vi "TraverseControl_High.vi"(0 "Mode":T3=enum."Read traverse position", 1 "Route Checking?":bool, 2 "Home":T2, 3 "Traverse Name":string, 5 "Extra command String":string, 6 "Work in Tunnel Coordinates":T1, 7 "Model       Roll      Pitch       Yaw (deg)":sgl[](array[numeric]) format="%#.2f", 9 "Final iteration of 3D_Trav Loop":bool=TRUE, 11 "Position input XYZ":sgl[](array[numeric])=[0.0, 0.0, 0.0] format="%.2f", 12 "Last Part of Move?":bool, 13 "Speed Factor":sgl=1.0 min=0.1 max=5 format="%.2f", 14 "Backlash Compensation?":bool=TRUE) -> (4 "Position Output XYZ":sgl[](array[numeric]) format="%.2f", 15 "Error String":string)   [LabVIEW 2017]
uses:
  Anemometry/Anemometry Sub Vis/Gen Trav/Trav_mode.ctl
  Anemometry/Anemometry Sub Vis/Controls/Home.ctl
  Anemometry/Anemometry Sub Vis/Controls/Tunnel_Coordinates.ctl
  Anemometry/Anemometry Sub Vis/Globals/Extra_Commands_Global.vi
  Anemometry/Anemometry Sub Vis/Globals/Trav_pos_global.vi
  Anemometry/Anemometry Sub Vis/Gen Trav/Route mapping/Route_mapping_global.vi
panel:
  out "Offset Array":sgl[](array[numeric])
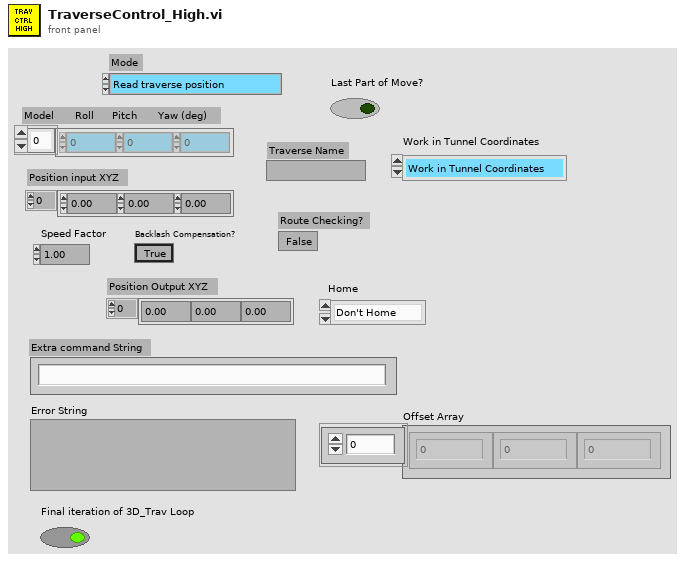
[diagram p1: front panel]
types:
  T1 = typedef "Tunnel_Coordinates.ctl" = enum16{"Work in Tunnel Coordinates", "Work in Model Coordinates"}
  T2 = typedef "Home.ctl" = enum16{"Don't Home", "Home  +X", "Home  -X", "Home  +Y", "Home  -Y", "Home  +Z", "Home  -Z"}
  T3 = typedef "Trav_mode.ctl" = enum16{"Move traverse", "Read traverse position", "Teach Position"}
  T4 = enum16{"To Traverse Coordinates", "To User Coordinates"}
  T5 = typedef "Axis.ctl" = enum16{"X Axis", "X Axis -ve", "Y Axis", "Y Axis -ve", "Z Axis", "Z Axis -ve"}
  T6 = typedef "Box_size.ctl" = cluster{"Max":sgl, "Min":sgl}[]
  T7 = typedef "Exclude_cluster.ctl" = cluster{"Sizes":T6, "Name":string, "Exclude Type":T8}
  T8 = typedef "Exclusion_type.ctl" = enum16{"Exclude completely", "Allow only vertical moves"}
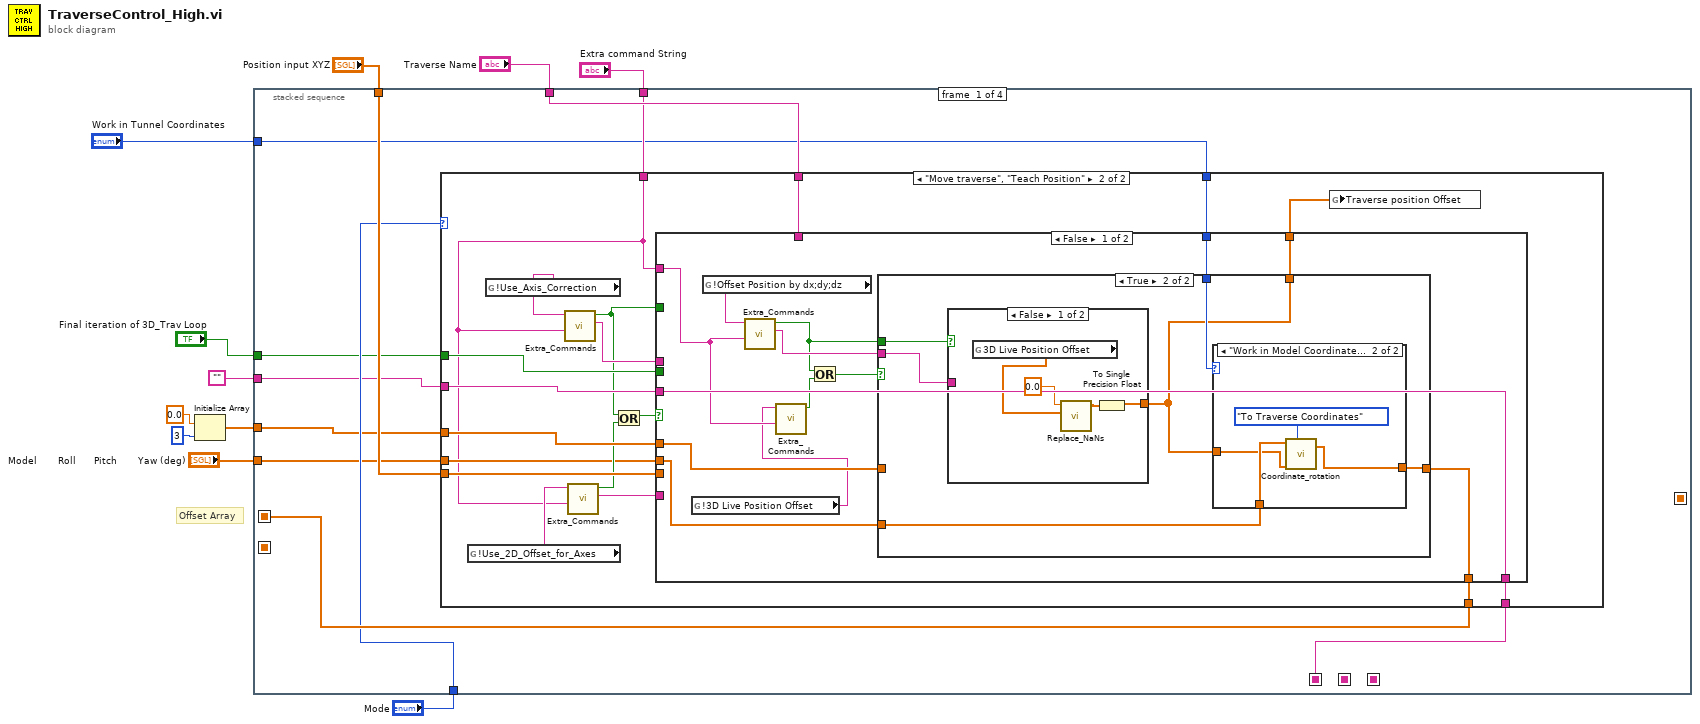
[diagram p0: block diagram]
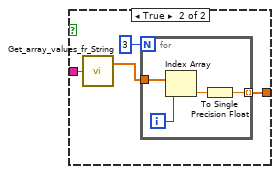
[diagram p4: hidden frame]
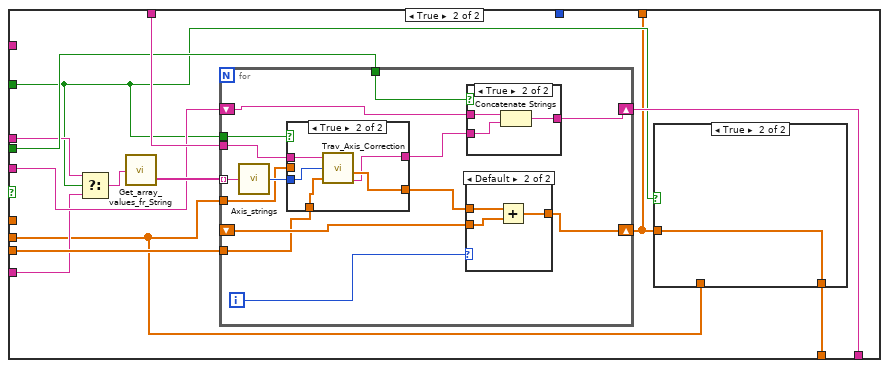
[diagram p6: hidden frame]
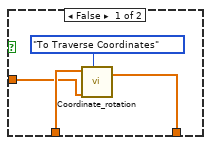
[diagram p7: hidden frame]
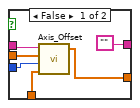
[diagram p8: hidden frame]
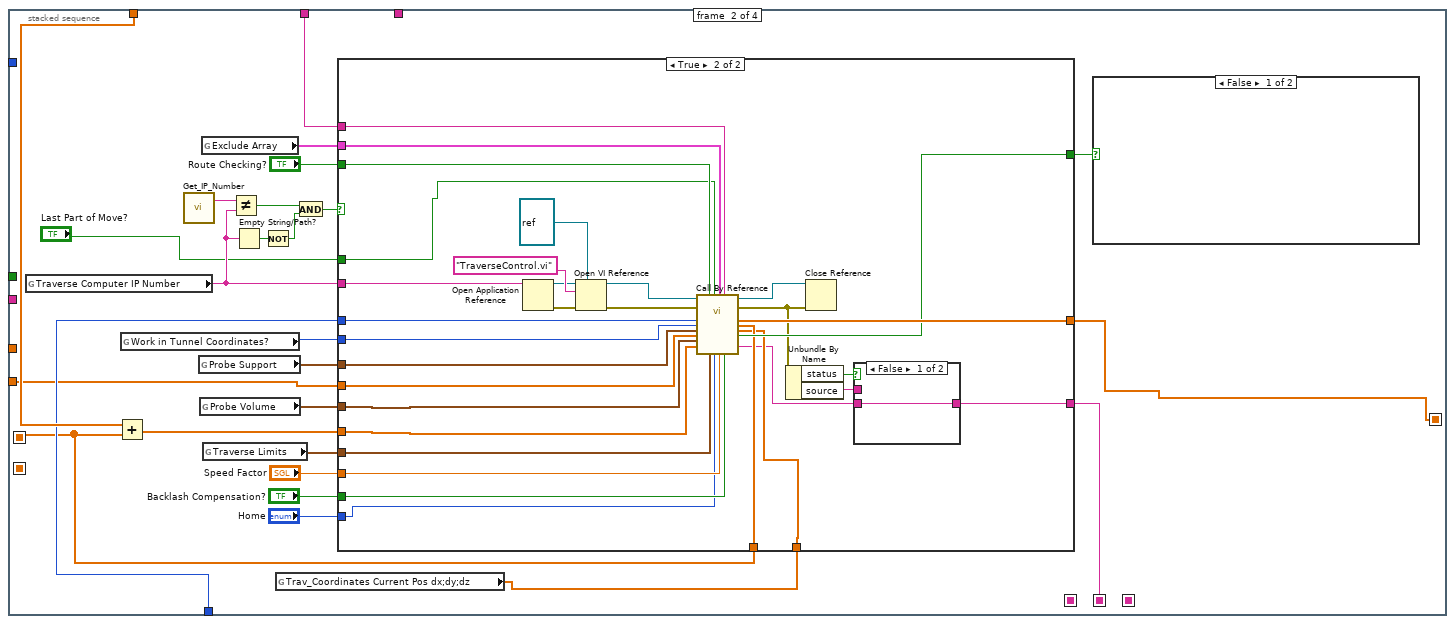
[diagram p11: hidden frame]
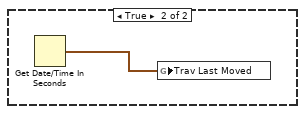
[diagram p12: hidden frame]
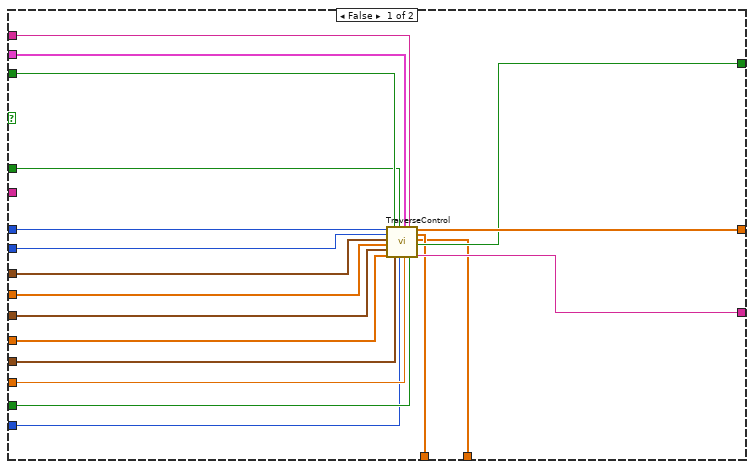
[diagram p13: hidden frame]
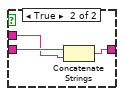
[diagram p14: hidden frame]
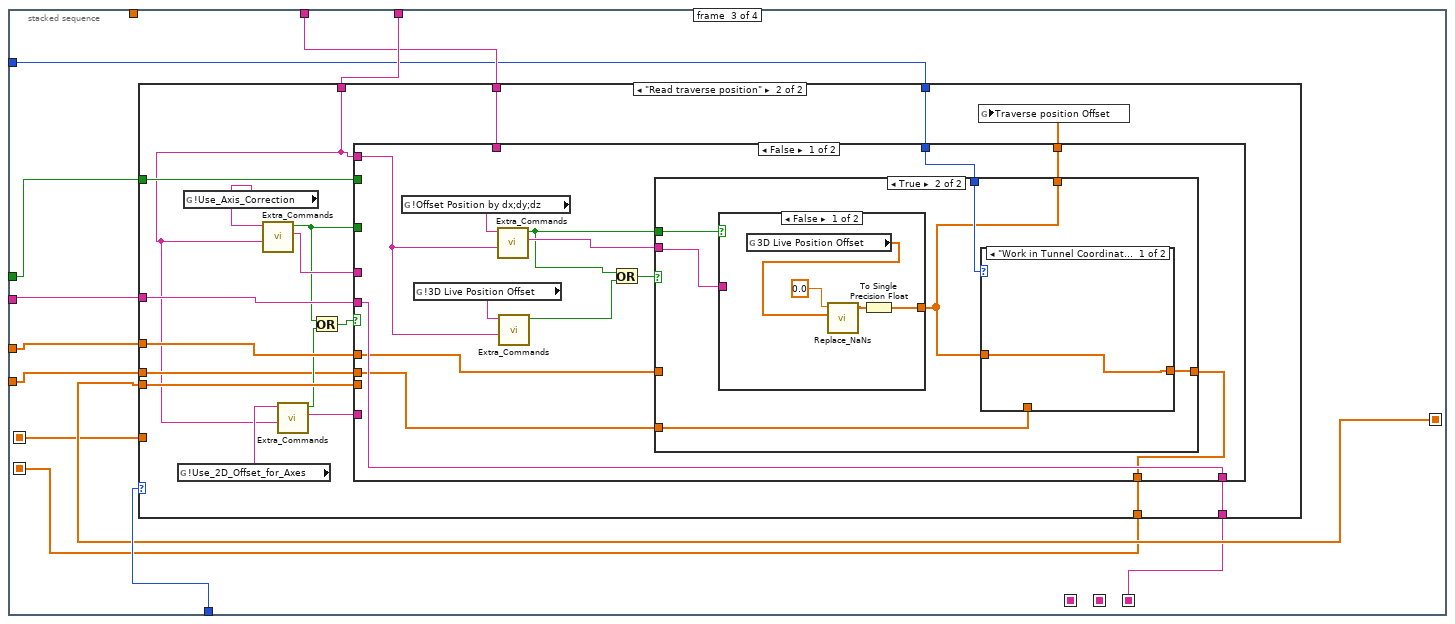
[diagram p15: hidden frame]
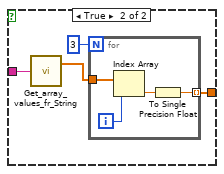
[diagram p18: hidden frame]
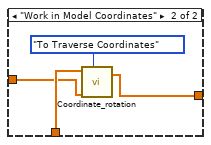
[diagram p19: hidden frame]
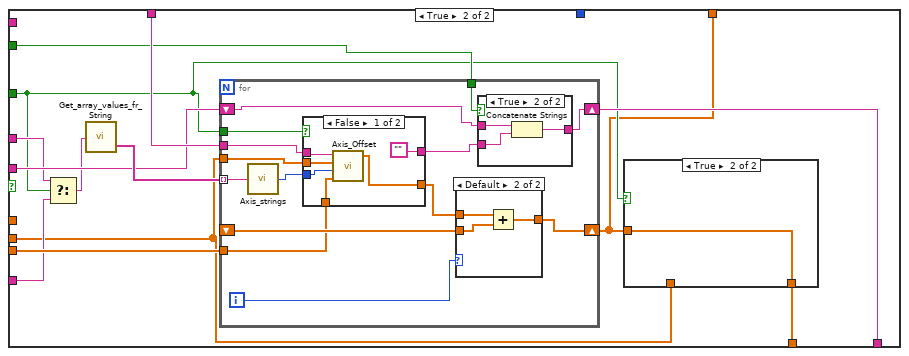
[diagram p20: hidden frame]
diagram:
  # "Offset Array"
  n1 = Initialize Array(sgl 0.0, 3 ("dimension size")) -> (w5:sgl[])
  n2 = stacked-sequence {
    seq-local: [_ w140 _ _] -> [_ _ w219 w337]
    seq-local: [w22 _ _ _] -> [_ w132 w215 _]
    seq-local: [w19 _ _ _] -> [_ _ _ w333]
    seq-local: [_ _ w217 _] -> [_ _ _ w332]
    seq-local: [_ _ w216 _] -> [_ _ _ w335]
    seq-local: [_ w135 _ _] -> [_ _ _ w334]
    tunnel: "Traverse Name" -> [w21 w139 w221 _]
    tunnel: "Position input XYZ" -> [w20 w138 _ _]
    tunnel: "Mode" -> [w17 w136 w223 _]
    tunnel: "Extra command String" -> [w18 _ w222 _]
    tunnel: w5 -> [w16 _ w218 _]
    tunnel: "" -> [w15 _ w220 _]
    tunnel: "Final iteration of 3D_Trav Loop" -> [w14 _ w214 _]
    tunnel: "Model       Roll      Pitch       Yaw (deg)" -> [w13 w133 w213 _]
    tunnel: "Work in Tunnel Coordinates" -> [w12 _ w212 _]
    frame #0 {
      n3 = case shown="\"Move traverse\", \"Teach Position\"" w17 {
        tunnel: [w23 w41] -> w22
        tunnel: w21 -> [_ w40]
        tunnel: w20 -> [_ w38]
        tunnel: [w24 w37] -> w19
        tunnel: w18 -> [_ w27]
        tunnel: w16 -> [w23 w36]
        tunnel: w15 -> [w24 w35]
        tunnel: w14 -> [_ w34]
        tunnel: w13 -> [_ w28]
        tunnel: w12 -> [_ w25]
        frame Default {
        }
        frame "Move traverse", "Teach Position" {
          n4 = global read "Extra_Commands_Global.vi" "!Use_2D_Offset_for_Axes"() -> (w33:string)
          n5 = global read "Extra_Commands_Global.vi" "!Use_Axis_Correction"() -> (w42:string)
          n6 = call "Extra_Commands.vi"("String to Search"=w27, "Command"=w42) -> ("String Value"=w39:string, "Command Found"=w30:bool)  [unwired: 1 in, 3 out]
          n7 = call "Extra_Commands.vi"("String to Search"=w27, "Command"=w33) -> ("String Value"=w29:string, "Command Found"=w32:bool)  [unwired: 1 in, 3 out]
          n8 = Or(x=w30, y=w32) -> (x .or. y?=w31:bool)
          n9 = case shown="False" w31 {
            tunnel: [w51 w82] -> w41
            tunnel: w38 -> [_ w90]
            tunnel: w40 -> [_ w91]
            tunnel: w39 -> [_ w86]
            tunnel: [w55 w87] -> w37
            tunnel: w35 -> [w55 w89]
            tunnel: w36 -> [w52 _]
            tunnel: w34 -> [_ w88]
            tunnel: w30 -> [_ w81]
            tunnel: w29 -> [_ w85]
            tunnel: w28 -> [w49 w83]
            tunnel: w27 -> [w44 _]
            tunnel: [w48 w80] -> w26
            tunnel: w25 -> [w50 _]
            frame False {
              n10 = global read "Extra_Commands_Global.vi" "!3D Live Position Offset"() -> (w43:string)
              n11 = global read "Extra_Commands_Global.vi" "!Offset Position by dx;dy;dz"() -> (w54:string)
              n12 = call "Extra_Commands.vi"("String to Search"=w44, "Command"=w54) -> ("String Value"=w53:string, "Command Found"=w45:bool)  [unwired: 1 in, 3 out]
              n13 = call "Extra_Commands.vi"("String to Search"=w44, "Command"=w43) -> ("Command Found"=w47:bool)  [unwired: 1 in, 4 out]
              n14 = Or(x=w45, y=w47) -> (x .or. y?=w46:bool)
              n15 = case shown="True" w46 {
                tunnel: w53 -> [_ w62]
                tunnel: [w56 w60] -> w51
                tunnel: w52 -> [w56 _]
                tunnel: w50 -> [_ w61]
                tunnel: w49 -> [_ w59]
                tunnel: [w56 w58] -> w48
                tunnel: w45 -> [_ w57]
                frame False {
                }
                frame True {
                  n16 = case shown="False" w57 {
                    tunnel: w62 -> [_ w69]
                    tunnel: [w64 w67] -> w58
                    frame False {
                      n17 = global read "Trav_pos_global.vi" "3D Live Position Offset"() -> (w63:sgl[])
                      n18 = call "Replace_NaNs.vi"("Array"=w63, "Replacement"=0.0) -> ("Array Out"=w65:dbl[])  [unwired: 9 in]
                      n19 = To Single Precision Float(number=w65) -> (single precision float=w64:sgl[])
                    }
                    frame True {
                      n20 = call "Get_array_values_fr_String.vi"("String Value"=w69) -> ("Numeric Array"=w68:dbl[])  [unwired: 1 out]
                      n21 = for {
                        N: 3 -> [_]
                        tunnel: w68 -> [w74]
                        tunnel: [w71] -> w67 mode=indexing
                        i -> [w73]
                        n22 = Index Array(array=w74, index=w73) -> (element=w72:dbl)
                        n23 = To Single Precision Float(number=w72) -> (single precision float=w71:sgl)
                      }
                    }
                  }
                  n24 = case shown="\"Work in Model Coordinates\"" w61 {
                    tunnel: w58 -> [w75 w76]
                    tunnel: w59 -> [_ w79]
                    tunnel: [w75 w78] -> w60
                    frame "Work in Tunnel Coordinates" {
                    }
                    frame "Work in Model Coordinates" {
                      n25 = call "Coordinate_rotation.vi"("Roll-Pitch-Yaw"=w79, "Input Position"=w76, "Mode"=T4."To Traverse Coordinates") -> ("Output Position"=w78:sgl[])  [unwired: 2 in, 1 out]
                    }
                  }
                }
              }
            }
            frame True {
              n26 = Select(t=w86, s=w81, f=w85) -> (s? t:f=w84:string)
              n27 = call "Get_array_values_fr_String.vi"("String Value"=w84) -> ("String array"=w92:string[])  [unwired: 1 out]
              n28 = for {
                tunnel: w92 -> [w111] mode=indexing
                tunnel: w91 -> [w104]
                tunnel: w90 -> [w102]
                shift-right: [w109] -> w80
                shift-left: _ -> [w110]
                shift-right: [w106] -> w87
                shift-left: w89 -> [w107]
                tunnel: w88 -> [w105]
                tunnel: w81 -> [w98]
                tunnel: w83 -> [w99]
                i -> [w108]
                n29 = call "Axis_strings.vi"("String"=w111) -> ("Enum"=w103:T5)
                n30 = case shown="True" w98 {
                  tunnel: w104 -> [w116 w122]
                  tunnel: w103 -> [w115 w121]
                  tunnel: w102 -> [w114 w120]
                  tunnel: [w117 w119] -> w101
                  tunnel: ["" w118] -> w100
                  tunnel: w99 -> [w112 _]
                  frame False {
                    n31 = call "Axis_Offset.vi"("Position In"=w114, "Axis"=w115, "Roll-Pitch-Yaw"=w112, "Traverse Name"=w116) -> ("Offset Array"=w117:sgl[])  [unwired: 2 out]
                  }
                  frame True {
                    n32 = call "Trav_Axis_Correction.vi"("Traverse Name"=w122, "Axis"=w121, "Position input XYZ"=w120) -> ("Offset Array"=w119:sgl[], "Error String"=w118:string)  [unwired: 2 out]
                  }
                }
                n33 = case shown="Default" w108 {
                  tunnel: w101 -> [w127 w130]
                  tunnel: w110 -> [_ w129]
                  tunnel: [w127 w128] -> w109
                  frame 0 {
                  }
                  frame Default {
                    n34 = Add(x=w130, y=w129) -> (x+y=w128:sgl[])
                  }
                }
                n35 = case shown="True" w105 {
                  tunnel: w100 -> [_ w126]
                  tunnel: w107 -> [w123 w125]
                  tunnel: [w123 w124] -> w106
                  frame False {
                  }
                  frame True {
                    n36 = Concatenate Strings(w125, w126) -> (w124:string)
                  }
                }
              }
              n37 = case shown="True" w81 {
                tunnel: w80 -> [w93 w97]
                tunnel: w83 -> [w96 _]
                tunnel: [w95 w97] -> w82
                frame False {
                  n38 = call "Coordinate_rotation.vi"("Roll-Pitch-Yaw"=w96, "Input Position"=w93, "Mode"=T4."To Traverse Coordinates") -> ("Output Position"=w95:sgl[])  [unwired: 2 in, 1 out]
                }
                frame True {
                }
              }
            }
          }
          n39 = global write "Trav_pos_global.vi" "Traverse position Offset"(w26) -> ()
        }
      }
    }
    frame #1 {
      n40 = global read "Trav_pos_global.vi" "Traverse Computer IP Number"() -> (w150:string)
      n41 = Add(x=w138, y=w132) -> (x+y=w137:sgl[])
      n42 = global read "Trav_pos_global.vi" "Work in Tunnel Coordinates?"() -> (w144:T1)
      n43 = call "Get_IP_Number.vi"() -> ("IP Number"=w156:string)  [unwired: 1 out]
      n44 = global read "Route_mapping_global.vi" "Probe Support"() -> (w143:T6)
      n45 = global read "Route_mapping_global.vi" "Probe Volume"() -> (w145:T6)
      n46 = global read "Route_mapping_global.vi" "Exclude Array"() -> (w147:T7[])
      n47 = global read "Route_mapping_global.vi" "Traverse Limits"() -> (w146:T6)
      n48 = Not Equal?(x=w156, y=w150) -> (x != y?=w149:bool)
      n49 = Empty String/Path?(string/path=w150) -> (empty?=w152:bool)
      n50 = Not(x=w152) -> (.not. x?=w151:bool)
      n51 = global read "Trav_pos_global.vi" "Trav_Coordinates Current Pos dx;dy;dz"() -> (w131:sgl[])
      n52 = And(x=w149, y=w151) -> (x .and. y?=w148:bool)
      n53 = case shown="True" w148 {
        tunnel: "Route Checking?" -> [w169 w207]
        tunnel: w139 -> [w168 w206]
        tunnel: [w175 w205] -> w140
        tunnel: [w176 w197] -> w135
        tunnel: "Backlash Compensation?" -> [w172 w204]
        tunnel: "Speed Factor" -> [w171 w203]
        tunnel: w137 -> [w174 w202]
        tunnel: w133 -> [w173 w201]
        tunnel: w136 -> [w170 w200]
        tunnel: w150 -> [_ w199]
        tunnel: w147 -> [w167 w198]
        tunnel: w146 -> [w166 w194]
        tunnel: w145 -> [w165 w195]
        tunnel: w144 -> [w164 w196]
        tunnel: w143 -> [w163 w193]
        tunnel: "Last Part of Move?" -> [w162 w192]
        tunnel: "Home" -> [w161 w191]
        tunnel: [w160 w190] -> w141
        tunnel: w132 -> [w159 w189]
        tunnel: w131 -> [w158 w188]
        frame False {
          n54 = call "TraverseControl.vi"("Mode"=w170, "Work in Tunnel Coordinates?"=w164, "Probe Support"=w163, "Model       Roll      Pitch       Yaw (deg)"=w173, "Probe Volume"=w165, "Position input XYZ"=w174, "Route Checking?"=w169, "Entire Space"=w166, "Last Part of Move?"=w162, "Home"=w161, "Exclude Array"=w167, "Speed Factor"=w171, "Traverse Name"=w168, "Backlash Compensation?"=w172, "Trav_Coordinates New Pos dx;dy;dz"=w159, "Trav_Coordinates Current Pos dx;dy;dz"=w158) -> ("Position Output XYZ"=w175:sgl[], "Moved?"=w160:bool, "Error String"=w176:string)  [unwired: 1 in]
        }
        frame True {
          n55 = Open Application Reference(11:w199) -> (0:w181:errorcluster, 3:w182:refnum<vi>)  [unwired: 2 in, 1 out]
          n56 = Open VI Reference(type specifier VI Refnum (for type only)=refnum<vi> refnum ("Scout Server"), application reference (local)=w182, vi path="TraverseControl.vi", error in (no error)=w181) -> (vi reference=w185:refnum<vi>, error out=w184:errorcluster)  [unwired: 2 out]
          n57 = call-by-ref "?"(reference=w185, error in=w184, "Mode"=w200, "Work in Tunnel Coordinates?"=w196, "Probe Support"=w193, "Model       Roll      Pitch       Yaw (deg)"=w201, "Probe Volume"=w195, "Position input XYZ"=w202, "Route Checking?"=w207, "Entire Space"=w194, "Last Part of Move?"=w192, "Home"=w191, "Exclude Array"=w198, "Speed Factor"=w203, "Traverse Name"=w206, "Backlash Compensation?"=w204, "Trav_Coordinates New Pos dx;dy;dz"=w189, "Trav_Coordinates Current Pos dx;dy;dz"=w188) -> (reference out=w183:refnum<vi>, error out=w180:errorcluster, "Position Output XYZ"=w205:sgl[], "Moved?"=w190:bool, "Error String"=w178:string)  [unwired: 1 in]
          n58 = Unbundle By Name(w180) -> ("status"=w179:bool, "source"=w177:string)
          n59 = Close Reference(reference=w183, error in (no error)=w180) -> ()  [unwired: 1 out]
          n60 = case shown="False" w179 {
            tunnel: [w208 w211] -> w197
            tunnel: w178 -> [w208 w210]
            tunnel: w177 -> [_ w209]
            frame False {
            }
            frame True {
              n61 = Concatenate Strings(w210, w209) -> (w211:string)
            }
          }
        }
      }
      n62 = case shown="False" w141 {
        frame False {
        }
        frame True {
          n63 = Get Date/Time In Seconds() -> (seconds since 1Jan1904=w157:timestamp)
          n64 = global write "Trav_pos_global.vi" "Trav Last Moved"(w157) -> ()
        }
      }
    }
    frame #2 {
      n65 = case shown="\"Read traverse position\"" w223 {
        tunnel: [w224 w242] -> w217
        tunnel: w221 -> [_ w241]
        tunnel: w219 -> [_ w239]
        tunnel: [w225 w238] -> w216
        tunnel: w222 -> [_ w228]
        tunnel: w218 -> [_ w237]
        tunnel: w220 -> [w225 w236]
        tunnel: w215 -> [w224 _]
        tunnel: w214 -> [_ w235]
        tunnel: w213 -> [_ w229]
        tunnel: w212 -> [_ w226]
        frame Default {
        }
        frame "Read traverse position" {
          n66 = global read "Extra_Commands_Global.vi" "!Use_2D_Offset_for_Axes"() -> (w234:string)
          n67 = global read "Extra_Commands_Global.vi" "!Use_Axis_Correction"() -> (w243:string)
          n68 = call "Extra_Commands.vi"("String to Search"=w228, "Command"=w243) -> ("String Value"=w240:string, "Command Found"=w231:bool)  [unwired: 1 in, 3 out]
          n69 = call "Extra_Commands.vi"("String to Search"=w228, "Command"=w234) -> ("String Value"=w230:string, "Command Found"=w232:bool)  [unwired: 1 in, 3 out]
          n70 = Or(x=w231, y=w232) -> (x .or. y?=w233:bool)
          n71 = case shown="False" w233 {
            tunnel: [w249 w284] -> w242
            tunnel: w239 -> [_ w291]
            tunnel: w241 -> [_ w292]
            tunnel: w240 -> [_ w287]
            tunnel: [w255 w290] -> w238
            tunnel: w236 -> [w255 w289]
            tunnel: w237 -> [w252 _]
            tunnel: w235 -> [_ w288]
            tunnel: w231 -> [_ w282]
            tunnel: w230 -> [_ w286]
            tunnel: w229 -> [w253 w283]
            tunnel: w228 -> [w247 _]
            tunnel: [w250 w281] -> w227
            tunnel: w226 -> [w251 _]
            frame False {
              n72 = global read "Extra_Commands_Global.vi" "!Offset Position by dx;dy;dz"() -> (w256:string)
              n73 = global read "Extra_Commands_Global.vi" "!3D Live Position Offset"() -> (w248:string)
              n74 = call "Extra_Commands.vi"("String to Search"=w247, "Command"=w256) -> ("String Value"=w254:string, "Command Found"=w244:bool)  [unwired: 1 in, 3 out]
              n75 = call "Extra_Commands.vi"("String to Search"=w247, "Command"=w248) -> ("Command Found"=w245:bool)  [unwired: 1 in, 4 out]
              n76 = Or(x=w244, y=w245) -> (x .or. y?=w246:bool)
              n77 = case shown="True" w246 {
                tunnel: [w257 w262] -> w249
                tunnel: w252 -> [w257 _]
                tunnel: w251 -> [_ w263]
                tunnel: w253 -> [_ w261]
                tunnel: [w257 w260] -> w250
                tunnel: w254 -> [_ w259]
                tunnel: w244 -> [_ w258]
                frame False {
                }
                frame True {
                  n78 = case shown="False" w258 {
                    tunnel: [w264 w269] -> w260
                    tunnel: w259 -> [_ w268]
                    frame False {
                      n79 = global read "Trav_pos_global.vi" "3D Live Position Offset"() -> (w266:sgl[])
                      n80 = call "Replace_NaNs.vi"("Array"=w266, "Replacement"=0.0) -> ("Array Out"=w265:dbl[])  [unwired: 9 in]
                      n81 = To Single Precision Float(number=w265) -> (single precision float=w264:sgl[])
                    }
                    frame True {
                      n82 = call "Get_array_values_fr_String.vi"("String Value"=w268) -> ("Numeric Array"=w270:dbl[])  [unwired: 1 out]
                      n83 = for {
                        N: 3 -> [_]
                        tunnel: w270 -> [w275]
                        tunnel: [w272] -> w269 mode=indexing
                        i -> [w274]
                        n84 = Index Array(array=w275, index=w274) -> (element=w273:dbl)
                        n85 = To Single Precision Float(number=w273) -> (single precision float=w272:sgl)
                      }
                    }
                  }
                  n86 = case shown="\"Work in Tunnel Coordinates\"" w263 {
                    tunnel: w260 -> [w276 w277]
                    tunnel: w261 -> [_ w280]
                    tunnel: [w276 w279] -> w262
                    frame "Work in Tunnel Coordinates" {
                    }
                    frame "Work in Model Coordinates" {
                      n87 = call "Coordinate_rotation.vi"("Roll-Pitch-Yaw"=w280, "Input Position"=w277, "Mode"=T4."To Traverse Coordinates") -> ("Output Position"=w279:sgl[])  [unwired: 2 in, 1 out]
                    }
                  }
                }
              }
            }
            frame True {
              n88 = Select(t=w287, s=w282, f=w286) -> (s? t:f=w285:string)
              n89 = call "Get_array_values_fr_String.vi"("String Value"=w285) -> ("String array"=w293:string[])  [unwired: 1 out]
              n90 = for {
                tunnel: w293 -> [w312] mode=indexing
                tunnel: w292 -> [w301]
                tunnel: w291 -> [w303]
                shift-right: [w310] -> w281
                shift-left: _ -> [w311]
                shift-right: [w307] -> w290
                shift-left: w289 -> [w308]
                tunnel: w288 -> [w306]
                tunnel: w282 -> [w300]
                tunnel: w283 -> [w299]
                i -> [w309]
                n91 = call "Axis_strings.vi"("String"=w312) -> ("Enum"=w302:T5)
                n92 = case shown="False" w300 {
                  tunnel: w301 -> [w317 w323]
                  tunnel: w302 -> [w316 w322]
                  tunnel: w303 -> [w315 w321]
                  tunnel: [w318 w320] -> w304
                  tunnel: ["" w319] -> w305
                  tunnel: w299 -> [w313 _]
                  frame False {
                    n93 = call "Axis_Offset.vi"("Position In"=w315, "Axis"=w316, "Roll-Pitch-Yaw"=w313, "Traverse Name"=w317) -> ("Offset Array"=w318:sgl[])  [unwired: 2 out]
                  }
                  frame True {
                    n94 = call "Trav_Axis_Correction.vi"("Traverse Name"=w323, "Axis"=w322, "Position input XYZ"=w321) -> ("Offset Array"=w320:sgl[], "Error String"=w319:string)  [unwired: 2 out]
                  }
                }
                n95 = case shown="Default" w309 {
                  tunnel: w304 -> [w328 w331]
                  tunnel: w311 -> [_ w330]
                  tunnel: [w328 w329] -> w310
                  frame 0 {
                  }
                  frame Default {
                    n96 = Add(x=w331, y=w330) -> (x+y=w329:sgl[])
                  }
                }
                n97 = case shown="True" w306 {
                  tunnel: w305 -> [_ w327]
                  tunnel: w308 -> [w324 w326]
                  tunnel: [w324 w325] -> w307
                  frame False {
                  }
                  frame True {
                    n98 = Concatenate Strings(w326, w327) -> (w325:string)
                  }
                }
              }
              n99 = case shown="True" w282 {
                tunnel: w281 -> [w297 w298]
                tunnel: w283 -> [w296 _]
                tunnel: [w295 w298] -> w284
                frame False {
                  n100 = call "Coordinate_rotation.vi"("Roll-Pitch-Yaw"=w296, "Input Position"=w297, "Mode"=T4."To Traverse Coordinates") -> ("Output Position"=w295:sgl[])  [unwired: 2 in, 1 out]
                }
                frame True {
                }
              }
            }
          }
          n101 = global write "Trav_pos_global.vi" "Traverse position Offset"(w227) -> ()
        }
      }
    }
    frame #3 {
      n102 = global write "Trav_pos_global.vi" "Trav_Coordinates Current Pos dx;dy;dz"(w332) -> ()
      n103 = Subtract(x=w337, y=w332) -> (x-y=→"Position Output XYZ":sgl[])
      n104 = Concatenate Strings(w333, w334, w335) -> (→"Error String":string)
      "Offset Array" <- w332
    }
  }
